vi "4-8 2D_array_Display.vi"() -> ()   [LabVIEW 2014]
doc: "------------------------------------\nAuther: Koji Ohashi\nCopyright (c) 2020 Japan LabVIEW Users Group, Volunteer members.\nThis VI is released under the MIT License.\nhttp://opensource.org/licenses/mit-license.php\n------------------------------------"
uses:
  <vilib>/Math Plots/3D Math Plots/3D Mesh/3D Mesh Datatype/3D Mesh Datatype.lvclass
  <vilib>/Math Plots/3D Math Plots/3D Mesh/3D Mesh Datatype/Public/Plot Helper (Matrix).vi
  <vilib>/Native 3D Graph/xcontrol/3DPC_SurfacePlot.xctl
  <vilib>/Math Plots/3D Math Plots/3D Mesh/3D Mesh XCtrl/3D Mesh.xctl
panel:
  out "Array":dbl[][](array[numeric])
  out "3D Graph":refnum<class "Base Datatype.lvclass">[](xcontrol)
  out "3D Mesh":refnum<class "3D Plot Datatype.lvclass">[](xcontrol)
  out "Intensity Graph":dbl[][](graph)
  # "Various display methods for a 2D array"
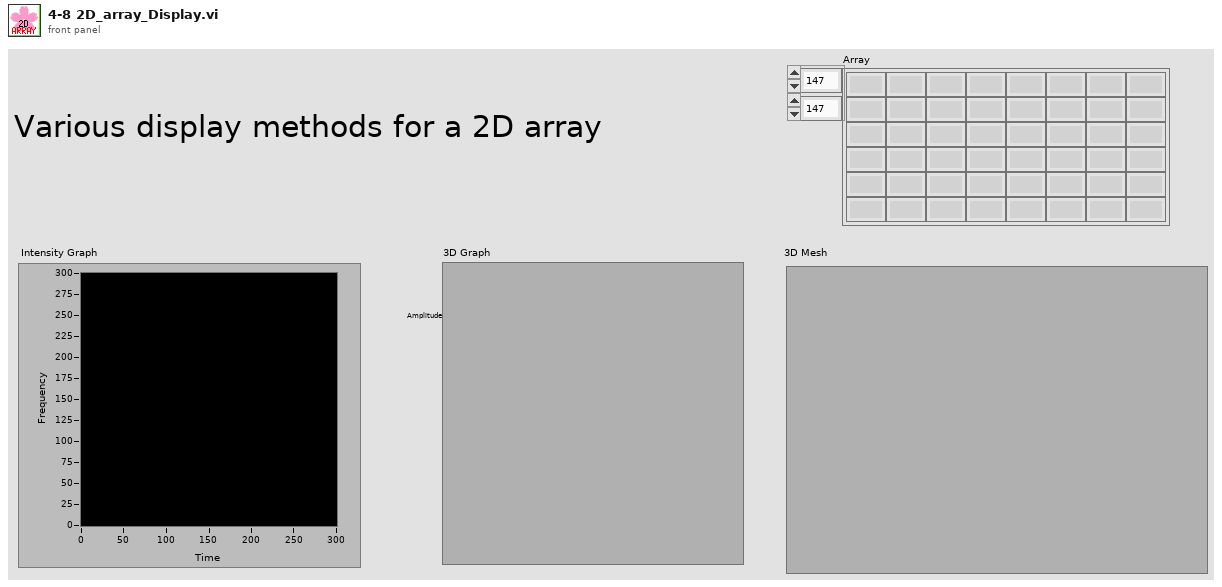
[diagram p1: front panel]
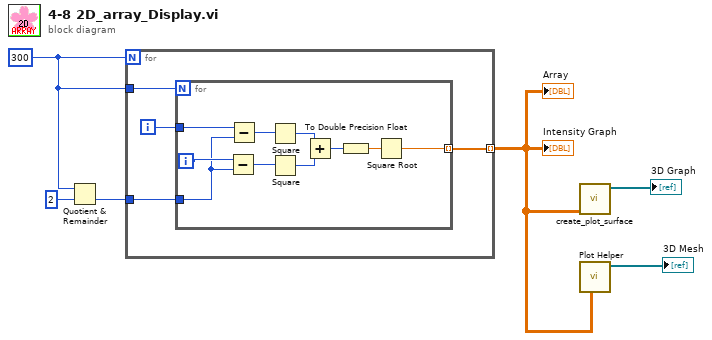
[diagram p0: block diagram]
diagram:
  w6 = 300
  n1 = Quotient & Remainder(x=w6, y=2) -> (floor(x/y)=w4:i32)  [unwired: 1 out]
  n2 = for {
    N: w6 -> [_]
    tunnel: w6 -> [w10]
    tunnel: w4 -> [w9]
    tunnel: [w7] -> w1 mode=indexing
    i -> [w8]
    n3 = for {
      N: w10 -> [_]
      tunnel: w9 -> [w18]
      tunnel: w8 -> [w20]
      tunnel: [w11] -> w7 mode=indexing
      i -> [w19]
      n4 = Subtract(x=w19, y=w18) -> (x-y=w16:i32)
      n5 = Subtract(x=w20, y=w18) -> (x-y=w17:i32)
      n6 = Square(x=w17) -> (x^2=w15:i32)
      n7 = Square(x=w16) -> (x^2=w14:i32)
      n8 = Add(x=w15, y=w14) -> (x+y=w13:i32)
      n9 = To Double Precision Float(number=w13) -> (double precision float=w12:dbl)
      n10 = Square Root(x=w12) -> (sqrt(x)=w11:dbl)
    }
  }
  "Intensity Graph" <- w1
  "Array" <- w1
  n11 = call <vilib>:"create_plot_surface.vi"("z matrix"=w1) -> ("plots out"=→"3D Graph":refnum<class "Base Datatype.lvclass">[])  [unwired: 4 in, 6 out]
  n12 = call-poly <vilib>:"Plot Helper.vi"("z matrix"=w1) -> ("3D Plot lvclass Array out"=→"3D Mesh":refnum<class "3D Plot Datatype.lvclass">[])  [unwired: 5 in, 5 out]
